vi "SetSEC.vi"(8 "error in (no error)":errorcluster, 10 "ecin100ns":u64=1) -> (0 "error out":errorcluster)   [LabVIEW 2015, in "ESLSCDLL.lvlib"]
uses:
  ESLSCDLL.lvlib
  Globals.vi
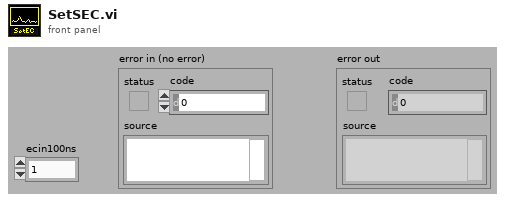
[diagram p1: front panel]
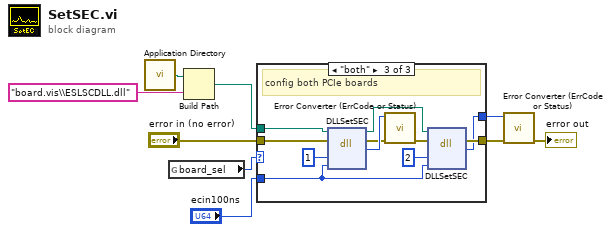
[diagram p0: block diagram]
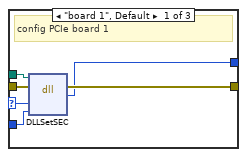
[diagram p2: hidden frame]
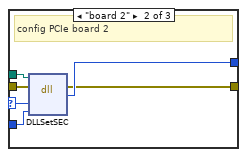
[diagram p3: hidden frame]
diagram:
  n1 = call <vilib>:"Application Directory.vi"() -> ("Application Directory"=w3:path)
  n2 = global read "Globals.vi" "board_sel"() -> (w4:enum32{"0", "board 1", "board 2", "both"})
  n3 = Build Path(base path=w3, name or relative path="board.vis\\ESLSCDLL.dll") -> (appended path=w1:path)
  n4 = case shown="\"both\"" w4 {
    selector: w4 -> [w14 w20 _]
    tunnel: "ecin100ns" -> [w15 w21 w30]
    tunnel: "error in (no error)" -> [w13 w17 w29]
    tunnel: [w12 w18 w25] -> w7
    tunnel: [w11 w19 w24] -> w5
    tunnel: w1 -> [w10 w16 w23]
    frame "board 1", Default {
      # "config PCIe board 1"
      n5 = dll-call lib="C:/ENTW/PCIE/LV64/board.vis/ESLSCDLL.dll" fn="DLLSetSEC" ("lwlscdll.dll:DLLSetTemp")(path in=w10, error in=w13, "drv"=w14, "ecin100ns"=w15) -> (error out=w12:errorcluster, "es_status_codes"=w11:i32)  [unwired: 3 in, 1 out]
    }
    frame "board 2" {
      # "config PCIe board 2"
      n6 = dll-call lib="C:/ENTW/PCIE/LV64/board.vis/ESLSCDLL.dll" fn="DLLSetSEC" ("lwlscdll.dll:DLLSetTemp")(path in=w16, error in=w17, "drv"=w20, "ecin100ns"=w21) -> (error out=w18:errorcluster, "es_status_codes"=w19:i32)  [unwired: 3 in, 1 out]
    }
    frame "both" {
      # "config both PCIe boards"
      n7 = dll-call lib="C:/ENTW/PCIE/LV64/board.vis/ESLSCDLL.dll" fn="DLLSetSEC" ("lwlscdll.dll:DLLSetTemp")(path in=w23, error in=w29, "drv"=u32 1, "ecin100ns"=w30) -> (path out=w22:path, error out=w27:errorcluster, "es_status_codes"=w28:i32)  [unwired: 3 in]
      n8 = call "Error Converter (ErrCode or Status).vi"("error in (no error)"=w27, "error code"=w28) -> ("error out"=w26:errorcluster)  [unwired: 9 in]
      n9 = dll-call lib="C:/ENTW/PCIE/LV64/board.vis/ESLSCDLL.dll" fn="DLLSetSEC" ("lwlscdll.dll:DLLSetTemp")(path in=w22, error in=w26, "drv"=u32 2, "ecin100ns"=w30) -> (error out=w25:errorcluster, "es_status_codes"=w24:i32)  [unwired: 3 in, 1 out]
    }
  }
  n10 = call "Error Converter (ErrCode or Status).vi"("error in (no error)"=w7, "error code"=w5) -> ("error out"=→"error out":errorcluster)  [unwired: 9 in]
